vi "iXonEMCCD_Single_Acquision.vi"() -> ()   [LabVIEW 2025]
uses:
  Library/atmcd32d.llb/TriggerMode_mode typedef.ctl
  Library/atmcd32d.llb/ReadMode_mode typedef.ctl
  Library/atmcd32d.llb/HSSpeed_type typedef.ctl
  Library/atmcd32d.llb/Error Code Enum typedef.ctl
  Library/atmcd32d.llb/Shutter_type typedef.ctl
  Library/atmcd32d.llb/Shutter_mode typedef.ctl
  Library/atmcd32d.llb/AcquisitionMode_mode typedef.ctl
panel:
  out "DLL error code 8":u32
  out "error out 8":errorcluster
  out "DLL error code 9":u32
  out "error out 9":errorcluster
  in  "error in (no error) 9":errorcluster
  out "DLL error code 7":u32
  out "error out 7":errorcluster
  out "DLL error code 6":u32
  out "error out 6":errorcluster
  out "DLL error code 5":u32
  out "error out 5":errorcluster
  out "DLL error code 2":u32
  out "error out 2":errorcluster
  out "DLL error code 3":u32
  out "error out 3":errorcluster
  in  "mode 2":T1=enum."Image"
  in  "Start Acquisition":bool
  in  "stop":bool
  out "DLL error code 13":u32
  out "error out 13":errorcluster
  out "error out 12":errorcluster
  out "DLL error code 12":u32
  out "kinetic":sgl format="%.2f"
  out "accumulate":sgl format="%.2f"
  out "exposure":sgl format="%.2f"
  in  "kinetic input":sgl format="%.2f"
  in  "accumulate input":sgl format="%.2f"
  in  "exposure input":sgl format="%.2f"
  out "error out 4":errorcluster
  out "DLL error code 4":u32
  out "error out 11":errorcluster
  out "DLL error code 11":u32
  in  "openingtime":i32
  in  "closingtime":i32
  in  "mode":T2
  in  "type 3":T3
  out "DLL error code 10":u32
  out "error out10":errorcluster
  in  "Number of Pulses":i32
  in  "channel 2":i32
  out "DLL error code 1":u32
  out "error out 1":errorcluster
  out "status":T4
  out "DLL error code 14":u32
  out "error out 14":errorcluster
  out "xpixels":i32
  out "ypixels":i32
  out "speed":sgl format="%.2f"
  in  "channel":i32
  in  "type 2":T5
  in  "index 2":i32
  in  "type":T5=enum."Conventional Amp"
  in  "index":i32
  in  "Read Mode":T1=enum."Image"
  out "DLL error code14":u32
  out "array 2":i32[](array[numeric])
  in  "Exposure Time (s)":sgl=1e-06 format="%.6f"
  in  "Trigger Mode":T6=enum."External Exposure (Bulb)"
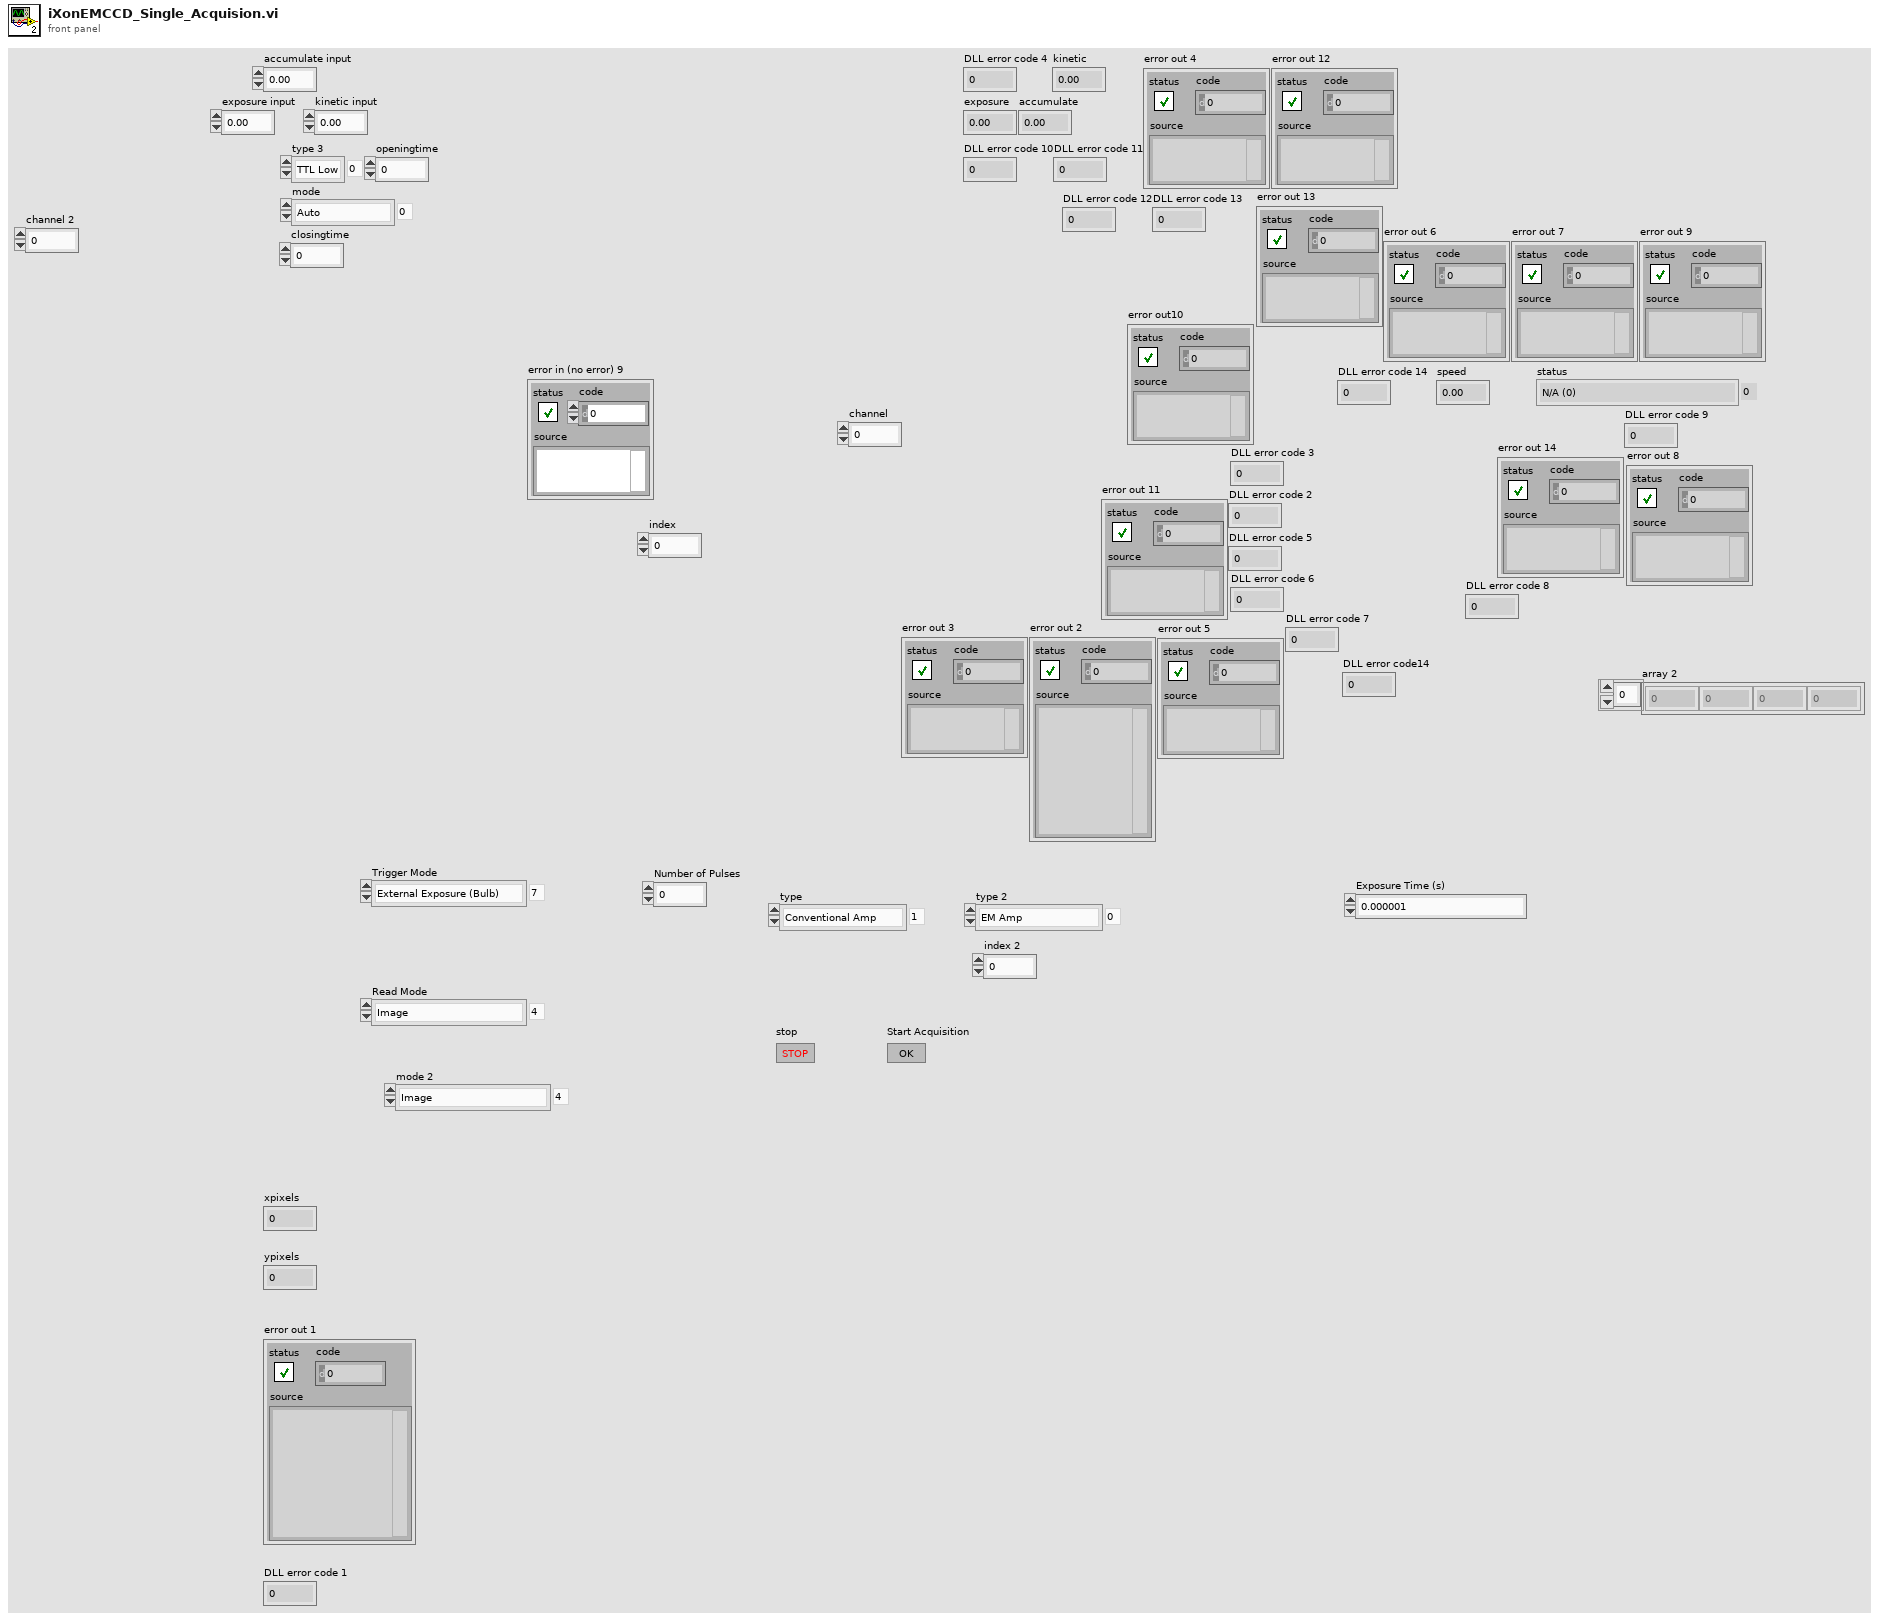
[diagram p1: front panel]
types:
  T1 = typedef "ReadMode_mode typedef.ctl" = enum16{"Full Vertical Binning", "Multi-Track", "Random-Track", "Single-Track", "Image"}
  T2 = typedef "Shutter_mode typedef.ctl" = enum16{"Auto", "Open", "Close", "N/A (3)", "Open FVB Series", "Open Any Series"}
  T3 = typedef "Shutter_type typedef.ctl" = enum16{"TTL Low", "TTL High"}
  T4 = typedef "Error Code Enum typedef.ctl" = enum32{"N/A (0)", "DRV_ERROR_CODES", "DRV_SUCCESS", "DRV_VXDNOTINSTALLED", "DRV_ERROR_SCAN", "DRV_ERROR_CHECK_SUM", "DRV_ERROR_FILELOAD", "DRV_UNKNOWN_FUNC", "DRV_ERROR_VXD_INIT", "DRV_ERROR_ADDRESS", "DRV_ERROR_PAGELOCK", "DRV_ERROR_PAGEUNLOCK", "DRV_ERROR_BOARDTEST", "DRV_ERROR_ACK", "DRV_ERROR_UP_FIFO", "DRV_ERROR_PATTERN", "N/A (16)", "DRV_ACQUISITION_ERRORS", "DRV_ACQ_BUFFER", "DRV_ACQ_DOWNFIFO_FULL", "DRV_PROC_UNKONWN_INSTRUCTION", "DRV_ILLEGAL_OP_CODE", "DRV_KINETIC_TIME_NOT_MET", "DRV_ACCUM_TIME_NOT_MET", "DRV_NO_NEW_DATA", "N/A (25)", "DRV_SPOOLERROR", "N/A (27)", "N/A (28)", "N/A (29)", "N/A (30)", "N/A (31)", "N/A (32)", "DRV_TEMPERATURE_CODES", "DRV_TEMPERATURE_OFF", "DRV_TEMPERATURE_NOT_STABILIZED", "DRV_TEMPERATURE_STABILIZED", "DRV_TEMPERATURE_NOT_REACHED", "DRV_TEMPERATURE_OUT_RANGE", "DRV_TEMPERATURE_NOT_SUPPORTED", "DRV_TEMPERATURE_DRIFT", "N/A (41)", "N/A (42)", "N/A (43)", "N/A (44)", "N/A (45)", "N/A (46)", "N/A (47)", "N/A (48)", "DRV_GENERAL_ERRORS", "DRV_INVALID_AUX", "DRV_COF_NOTLOADED", "DRV_FPGAPROG", "DRV_FLEXERROR", "DRV_GPIBERROR", "N/A (55)", "N/A (56)", "N/A (57)", "N/A (58)", "N/A (59)", "N/A (60)", "N/A (61)", "N/A (62)", "N/A (63)", "DRV_DATATYPE", "DRV_DRIVER_ERRORS", "DRV_P1INVALID", "DRV_P2INVALID", "DRV_P3INVALID", "DRV_P4INVALID", "DRV_INIERROR", "DRV_COFERROR", "DRV_ACQUIRING", "DRV_IDLE", "DRV_TEMPCYCLE", "DRV_NOT_INITIALIZED", "DRV_P5INVALID", "DRV_P6INVALID", "DRV_INVALID_MODE", "DRV_INVALID_FILTER", "DRV_I2CERRORS", "DRV_I2CDEVNOTFOUND", "DRV_I2CTIMEOUT", "DRV_P7INVALID", "N/A (84)", "N/A (85)", "N/A (86)", "N/A (87)", "N/A (88)", "N/A (89)", "DRV_IOCERROR", "DRV_VRMVERSIONERROR"}
  T5 = typedef "HSSpeed_type typedef.ctl" = enum16{"EM Amp", "Conventional Amp"}
  T6 = typedef "TriggerMode_mode typedef.ctl" = enum16{"Internal", "External", "N/A (2)", "N/A (3)", "N/A (4)", "N/A (5)", "External Start", "External Exposure (Bulb)", "N/A (8)", "External FVB EM", "Software", "N/A (11)", "External Charge Shifting"}
  T7 = typedef "AcquisitionMode_mode typedef.ctl" = enum16{"Reserved (0)", "Single Scan", "Accumulate", "Kinetics", "Fast Kinetics", "Run Till Abort", "Reserved (6)", "Reserved (7)", "Reserved (8)", "Time Delayed Integration"}
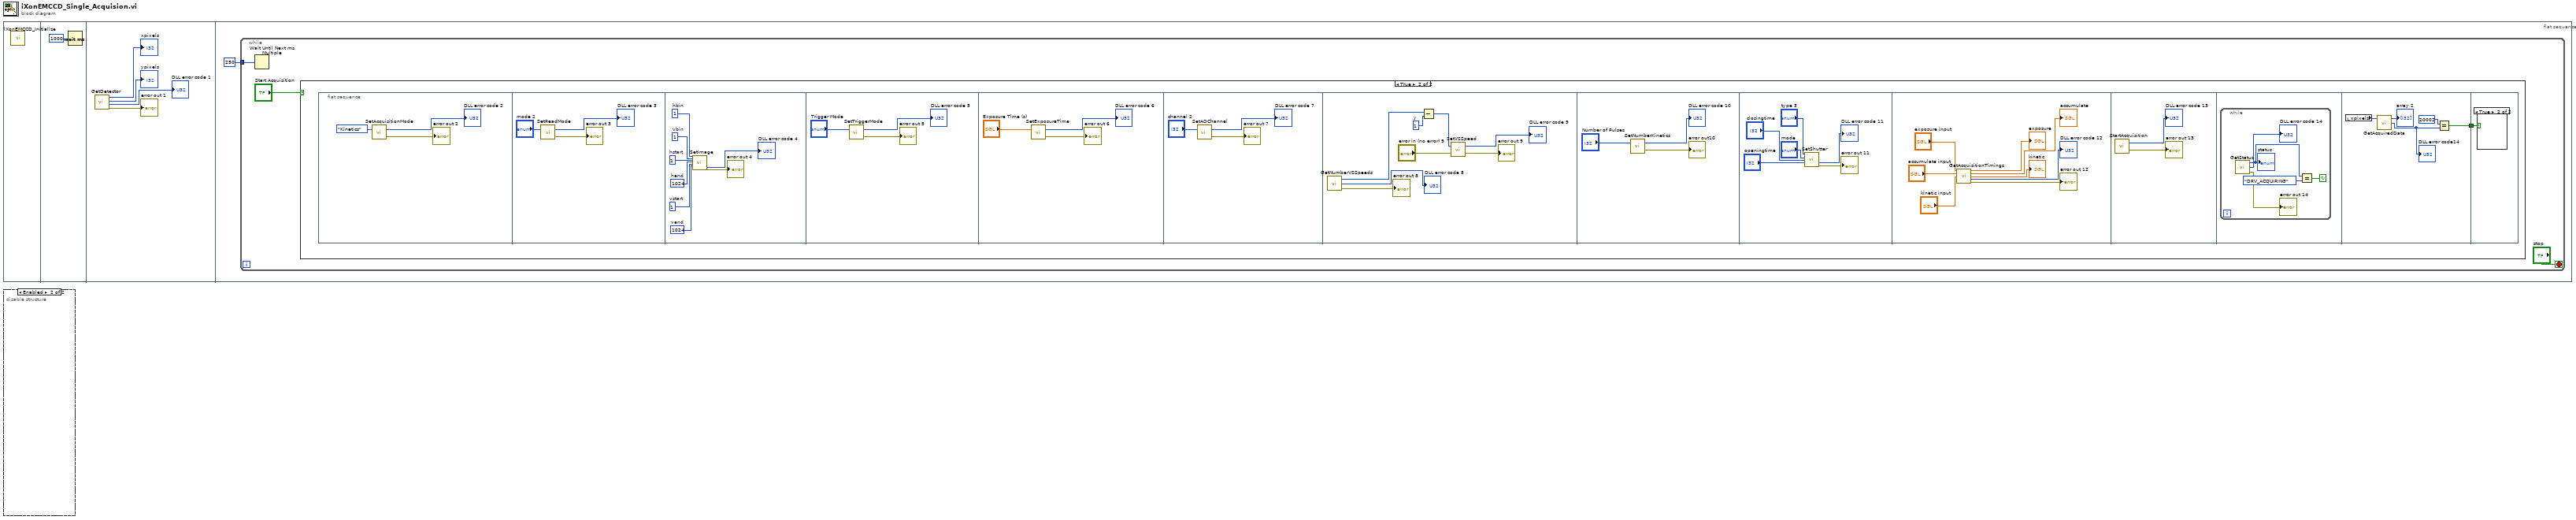
[diagram p0: block diagram]
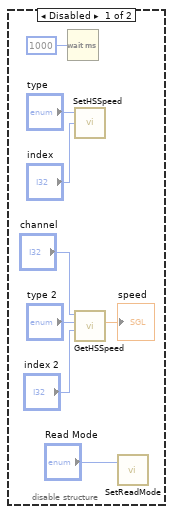
[diagram p2: hidden frame]
diagram:
  n1 = flat-sequence {
    frame #0 {
      n2 = call "iXonEMCCD_Initialize.vi"() -> ()  [unwired: 12 in]
    }
    frame #1 {
      n3 = Wait (ms)(milliseconds to wait=u32 1000) -> ()  [unwired: 1 out]
    }
    frame #2 {
      n4 = call "GetDetector.vi"() -> ("error out"=→"error out 1":errorcluster, "DLL error code"=→"DLL error code 1":u32, "ypixels"=→"ypixels":i32, "xpixels"=→"xpixels":i32)  [unwired: 4 in]
    }
    frame #3 {
      n5 = while {
        tunnel: 250 -> [w9]
        stop <- "stop" stop-if-true
        n6 = Wait Until Next ms Multiple(millisecond multiple=w9) -> ()  [unwired: 1 out]
        n7 = case shown="True" "Start Acquisition" {
          frame False {
          }
          frame True {
            n8 = flat-sequence {
              tunnel: [w66] -> w10
              tunnel: w10 -> [w71]
              frame #0 {
                n9 = call "SetAcquisitionMode.vi"("mode"=AcquisitionMode_mode_typedef."Kinetics") -> ("error out"=→"error out 2":errorcluster, "DLL error code"=→"DLL error code 2":u32)  [unwired: 1 in]
              }
              frame #1 {
                n10 = call "SetReadMode.vi"("mode"="mode 2") -> ("error out"=→"error out 3":errorcluster, "DLL error code"=→"DLL error code 3":u32)  [unwired: 1 in]
              }
              frame #2 {
                w19 = 1024  # vend
                w20 = 1  # vstart
                w21 = 1024  # hend
                w22 = 1  # hstart
                w23 = 1  # vbin
                w24 = 1  # hbin
                n11 = call "SetImage.vi"("hbin"=w24, "vbin"=w23, "hstart"=w22, "hend"=w21, "vstart"=w20, "vend"=w19) -> ("DLL error code"=→"DLL error code 4":u32, "error out"=→"error out 4":errorcluster)  [unwired: 20 in]
              }
              frame #3 {
                n12 = call "SetTriggerMode.vi"("mode"="Trigger Mode") -> ("error out"=→"error out 5":errorcluster, "DLL error code"=→"DLL error code 5":u32)  [unwired: 1 in]
              }
              frame #4 {
                n13 = call "SetExposureTime.vi"("time"="Exposure Time (s)") -> ("error out"=→"error out 6":errorcluster, "DLL error code"=→"DLL error code 6":u32)  [unwired: 1 in]
              }
              frame #5 {
                n14 = call "SetADChannel.vi"("channel"="channel 2") -> ("error out"=→"error out 7":errorcluster, "DLL error code"=→"DLL error code 7":u32)  [unwired: 1 in]
              }
              frame #6 {
                w40 = 1  # y
                n15 = call "GetNumberVSSpeeds.vi"() -> ("error out"=→"error out 8":errorcluster, "DLL error code"=→"DLL error code 8":u32, "number"=w41:i32)  [unwired: 3 in]
                n16 = Subtract(x=w41, y=w40) -> (x-y=w39:i32)
                n17 = call "SetVSSpeed.vi"("error in (no error)"="error in (no error) 9", "index"=w39) -> ("error out"=→"error out 9":errorcluster, "DLL error code"=→"DLL error code 9":u32)
              }
              frame #7 {
                n18 = call "SetNumberKinetics.vi"("number"="Number of Pulses") -> ("error out"=→"error out10":errorcluster, "DLL error code"=→"DLL error code 10":u32)  [unwired: 1 in]
              }
              frame #8 {
                n19 = call "SetShutter.vi"("type"="type 3", "mode"="mode", "closingtime"="closingtime", "openingtime"="openingtime") -> ("DLL error code"=→"DLL error code 11":u32, "error out"=→"error out 11":errorcluster)  [unwired: 10 in]
              }
              frame #9 {
                n20 = call "GetAcquisitionTimings.vi"("exposure input"="exposure input", "accumulate input"="accumulate input", "kinetic input"="kinetic input") -> ("exposure"=→"exposure":sgl, "accumulate"=→"accumulate":sgl, "kinetic"=→"kinetic":sgl, "DLL error code"=→"DLL error code 12":u32, "error out"=→"error out 12":errorcluster)  [unwired: 8 in]
              }
              frame #10 {
                n21 = call "StartAcquisition.vi"() -> ("error out"=→"error out 13":errorcluster, "DLL error code"=→"DLL error code 13":u32)  [unwired: 2 in]
              }
              frame #11 {
                n22 = while {
                  stop <- w61 continue-if-true
                  n23 = call "GetStatus.vi"() -> ("error out"=→"error out 14":errorcluster, "DLL error code"=→"DLL error code 14":u32, "status"=w63:T4)  [unwired: 3 in]
                  "status" <- w63
                  n24 = Equal?(x=w63, y=Error_Code_Enum_typedef."DRV_ACQUIRING") -> (x = y?=w61:bool)
                }
              }
              frame #12 {
                n25 = local read "xpixels"() -> (w70:i32)
                n26 = call "GetAcquiredData.vi"("size"=w70) -> ("DLL error code"=w68:u32, "array"=→"array 2":i32[])  [unwired: 2 in, 1 out]
                "DLL error code14" <- w68
                n27 = Equal?(x=u32 20002, y=w68) -> (x = y?=w66:bool)
              }
              frame #13 {
                n28 = case shown="True" w71 {
                  frame False {
                  }
                  frame True {
                  }
                }
              }
            }
          }
        }
      }
    }
  }
  n29 = disable-structure shown="Enabled" {
    frame Disabled {
      n30 = Wait (ms)(milliseconds to wait=u32 1000) -> ()  [unwired: 1 out]
      n31 = call "SetHSSpeed.vi"("index"="index", "type"="type") -> ()  [unwired: 2 in, 2 out]
      n32 = call "GetHSSpeed.vi"("index"="index 2", "type"="type 2", "channel"="channel") -> ("speed"=→"speed":sgl)  [unwired: 2 in, 2 out]
      n33 = call "SetReadMode.vi"("mode"="Read Mode") -> ()  [unwired: 1 in, 2 out]
    }
    frame Enabled {
    }
  }
